vi "Ro(N).vi"(0 "Nкр MW":dbl, 5 "Nнач MW":dbl, 7 "Брой ГЦП":dbl, 9 "dRoN %":dbl format="%#_6e", 10 "stop":bool, 11 "dRoH2O %":dbl format="%#_6e", 12 "dRoXE %":dbl format="%#_6e", 15 "dRo %":dbl format="%#_6f") -> (4 "∆Ro(N) %":dbl format="%#_3g", 6 "∆Ro(N) beta":dbl format="%#_3g")   [LabVIEW 2023]
panel:
  out "date/time string":string
  in  "dRoXE %":dbl format="%#_6e"
  in  "dRoH2O %":dbl format="%#_6e"
  in  "dRoN %":dbl format="%#_6e"
  out "∆N(Ro) %":dbl format="%#_4f"
  out "∆N(Ro) MW":dbl format="%#_3f"
  out "C / MW":dbl format="%#_3e"
  out "ГЦП":dbl
  # "Всички коефициенти и ефекти на реактивност, отчетени от Албум НФХ или Приложение 4, се заместват във формулите със своя знак (+, -)!"
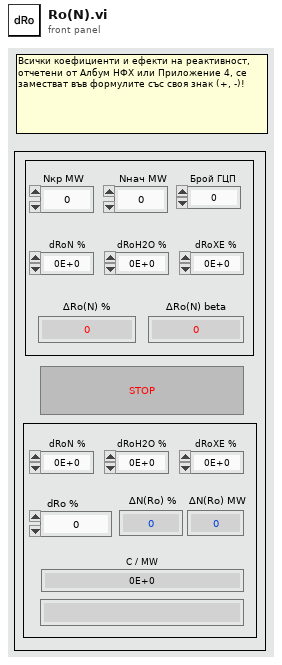
[diagram p1: front panel]
types:
  T1 = enum16{"Брой работещи ГЦП", "Пресмятане на темп. коефициенти", "Пресмятане на dRo(dN) ", "Пресмятане на dN(dRo)"}
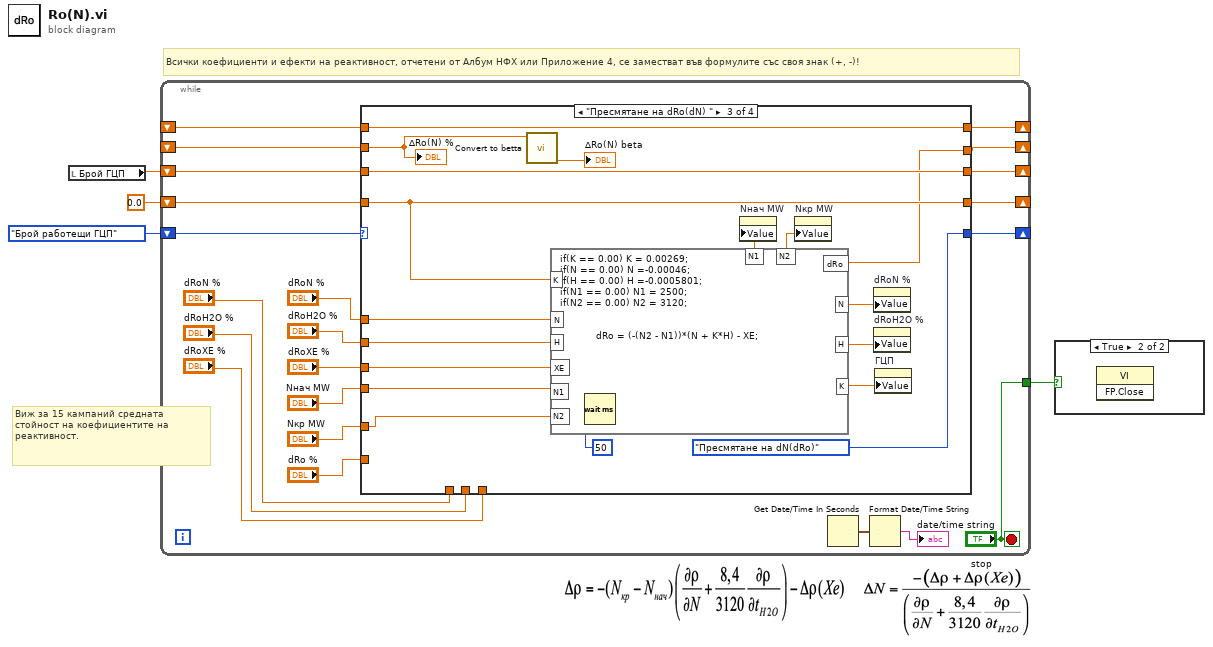
[diagram p0: block diagram]
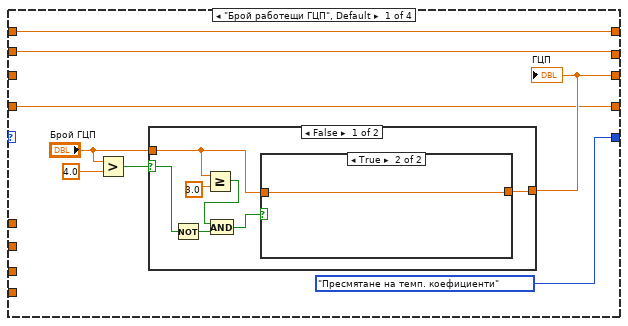
[diagram p3: hidden frame]
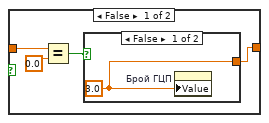
[diagram p4: hidden frame]
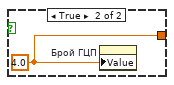
[diagram p5: hidden frame]
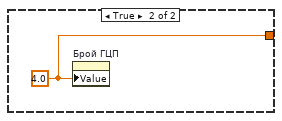
[diagram p6: hidden frame]
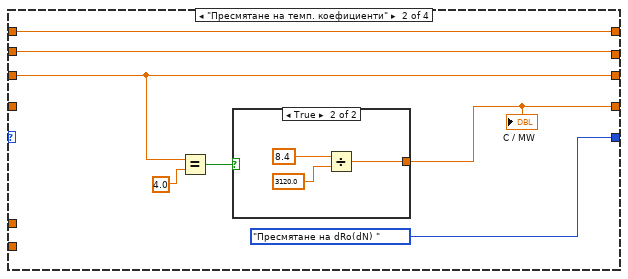
[diagram p7: hidden frame]
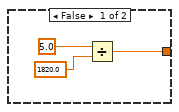
[diagram p8: hidden frame]
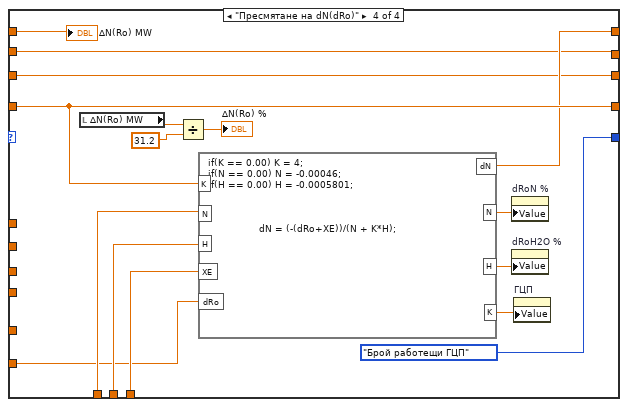
[diagram p9: hidden frame]
diagram:
  # "Виж за 15 кампаний средната стойност на коефициентите на \nреактивност."
  # "Всички коефициенти и ефекти на реактивност, отчетени от Албум НФХ или Приложение 4, се заместват във формулите със своя знак (+, -)!"
  n1 = local read "Брой ГЦП"() -> (w2:dbl)
  n2 = while {
    shift-right: [w26] -> _
    shift-left: w2 -> [w24]
    shift-right: [w23] -> _
    shift-left: T1."Брой работещи ГЦП" -> [w25]
    shift-right: [w22] -> _
    shift-left: 0.0 -> [w21]
    shift-right: [w20] -> _
    shift-left: _ -> [w19]
    shift-right: [w18] -> _
    shift-left: _ -> [w17]
    tunnel: ["stop"] -> w1
    stop <- "stop" stop-if-true
    n3 = case shown="\"Пресмятане на dRo(dN) \"" w25 {
      tunnel: [w30 w55 w80 w92] -> w26
      tunnel: w24 -> [_ w55 w80 w92]
      tunnel: [T1."Пресмятане на темп. коефициенти" T1."Пресмятане на dRo(dN) " T1."Пресмятане на dN(dRo)" T1."Брой работещи ГЦП"] -> w23
      tunnel: [w29 w52 w79 w96] -> w22
      tunnel: w21 -> [w29 _ w79 w96]
      tunnel: "dRoXE %" -> [_ _ w71 _]
      tunnel: "dRoH2O %" -> [_ _ w72 _]
      tunnel: "dRoN %" -> [_ _ w73 _]
      tunnel: "Nнач MW" -> [_ _ w70 _]
      tunnel: "Nкр MW" -> [_ _ w69 _]
      tunnel: "dRo %" -> [_ _ _ w84]
      tunnel: [w27 w51 w77 w93] -> w20
      tunnel: w19 -> [w27 w51 w75 w93]
      tunnel: [w28 w50 w76 w94] -> w18
      tunnel: w17 -> [w28 w50 w76 w91]
      tunnel: "dRoXE %" -> [_ _ _ w85]
      tunnel: "dRoH2O %" -> [_ _ _ w86]
      tunnel: "dRoN %" -> [_ _ _ w87]
      frame "Брой работещи ГЦП", Default {
        n4 = Greater?(x="Брой ГЦП", y=4.0) -> (0:w34:bool)
        n5 = case shown="False" w34 {
          selector: w34 -> [w37 _]
          tunnel: "Брой ГЦП" -> [w40 _]
          tunnel: [w35 w49] -> w30
          frame False {
            n6 = Not(x=w37) -> (.not. x?=w36:bool)
            n7 = Greater Or Equal?(x=w40, y=3.0) -> (x >= y?=w39:bool)
            n8 = And(x=w39, y=w36) -> (x .and. y?=w38:bool)
            n9 = case shown="True" w38 {
              tunnel: w40 -> [w45 w48]
              tunnel: [w42 w48] -> w35
              frame False {
                n10 = Equal?(x=w45, y=0.0) -> (x = y?=w43:bool)
                n11 = case shown="False" w43 {
                  tunnel: [w46 w47] -> w42
                  frame False {
                    w46 = 3.0 ("Брой ГЦП")
                    n12 = property on="Брой ГЦП" class="DigNum (strict)"("Value"=w46) -> ()  [unwired: 2 in, 2 out]
                  }
                  frame True {
                    w47 = 4.0 ("ГЦП")
                    n13 = property on="Брой ГЦП" class="DigNum (strict)"("Value"=w47) -> ()  [unwired: 2 in, 2 out]
                  }
                }
              }
              frame True {
              }
            }
          }
          frame True {
            w49 = 4.0 ("Брой ГЦП")
            n14 = property on="Брой ГЦП" class="DigNum (strict)"("Value"=w49) -> ()  [unwired: 2 in, 2 out]
          }
        }
        "ГЦП" <- w30
      }
      frame "Пресмятане на темп. коефициенти" {
        n15 = Equal?(x=w55, y=4.0) -> (x = y?=w54:bool)
        n16 = case shown="True" w54 {
          tunnel: [w57 w60] -> w52
          frame False {
            n17 = Divide(x=5.0, y=1820.0) -> (x/y=w57:dbl)
          }
          frame True {
            n18 = Divide(x=8.4, y=3120.0) -> (x/y=w60:dbl)
          }
        }
        "C / MW" <- w52
      }
      frame "Пресмятане на dRo(dN) " {
        # "Инициализира на първата интерация"
        n19 = call "Convert to betta.vi"("Ro %"=w75) -> ("Ro betta"=→"∆Ro(N) beta":dbl)  [unwired: 9 in]
        n20 = formula code="if(K == 0.00) K = 0.00269; \nif(N == 0.00) N =-0.00046;\nif(H == 0.00) H =-0.0005801;\nif(N1 == 0.00) N1 = 2500; \nif(N2 == 0.00) N2 = 3120; \n\n\n            dRo = (-(N2 - N1))*(N + K*H) - XE;"("N2"=w69, "N1"=w70, "XE"=w71, "H"=w72, "N"=w73, "K"=w79) -> ("dRo"=w77:dbl, "H"=w67:dbl, "N"=w68:dbl, "K"=w66:dbl, "N1"=w65:dbl, "N2"=w64:dbl)
        n21 = Wait (ms)(milliseconds to wait=u32 50) -> ()  [unwired: 1 out]
        n22 = property on="Nнач MW" class="DigNum (strict)"("Value"=w65) -> ()  [unwired: 2 in, 2 out]
        n23 = property on="Nкр MW" class="DigNum (strict)"("Value"=w64) -> ()  [unwired: 2 in, 2 out]
        n24 = property on="dRoN %" class="DigNum (strict)"("Value"=w68) -> ()  [unwired: 2 in, 2 out]
        n25 = property on="dRoH2O %" class="DigNum (strict)"("Value"=w67) -> ()  [unwired: 2 in, 2 out]
        n26 = property on="ГЦП" class="DigNum (strict)"("Value"=w66) -> ()  [unwired: 2 in, 2 out]
        "∆Ro(N) %" <- w75
      }
      frame "Пресмятане на dN(dRo)" {
        # "Инициализира на първата интерация на dRo(dN)"
        n27 = local read "∆N(Ro) MW"() -> (w90:dbl)
        n28 = Divide(x=w90, y=31.2) -> (x/y=→"∆N(Ro) %":dbl)
        n29 = formula code="if(K == 0.00) K = 4; \nif(N == 0.00) N = -0.00046;\nif(H == 0.00) H = -0.0005801; \n\n\n\n                 dN = (-(dRo+XE))/(N + K*H);"("XE"=w85, "H"=w86, "N"=w87, "K"=w96, "dRo"=w84) -> ("dN"=w94:dbl, "N"=w83:dbl, "H"=w82:dbl, "K"=w81:dbl)
        n30 = property on="dRoN %" class="DigNum (strict)"("Value"=w83) -> ()  [unwired: 2 in, 2 out]
        n31 = property on="dRoH2O %" class="DigNum (strict)"("Value"=w82) -> ()  [unwired: 2 in, 2 out]
        n32 = property on="ГЦП" class="DigNum (strict)"("Value"=w81) -> ()  [unwired: 2 in, 2 out]
        "∆N(Ro) MW" <- w91
      }
    }
    n33 = Get Date/Time In Seconds() -> (seconds since 1Jan1904=w6:timestamp)
    n34 = Format Date/Time String(seconds (now)=w6) -> (date/time string=→"date/time string":string)  [unwired: 2 in]
  }
  n35 = case shown="True" w1 {
    frame False {
    }
    frame True {
      n36 = invoke class="VI" method="FP.Close"() -> ()  [unwired: 3 in, 3 out]
    }
  }
